vi "Test-Main.vi"   [LabVIEW 2017]
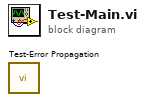
[diagram p0: block diagram]
diagram:
  n1 = call "Test-Error Propagation.vi"() -> ()  [unwired: 12 in]
